vi "ResonanceAnalyzer_for_week7.vi"() -> ()   [LabVIEW 2014]
uses:
  <vilib>/imath/engines/lvmath/Plug In/_Char/NIMS_CH_character datatype.ctl
  <vilib>/imath/engines/lvmath2/RunTimeEngine/Managers/WorkSpace/UID Generator.vi
  <vilib>/imath/engines/lvmath2/RunTimeEngine/RunTimeType/NIMS_RunTimeType_From StrictType (excl LVString).vi
  <instcachedir>/0/NIMS_RunTimeType_From StrictType (excl LVString)_15A5391EEA9C4AACB9955AC755B83D29.lvgen/NIMS_RunTimeType_From StrictType (excl LVString)_15A5391EEA9C4AACB9955AC755B83D29_000.vi
  <vilib>/imath/engines/lvmath2/RunTimeEngine/LocalVariableDefStatement/MC_LocalVariableDefStatement_Display.vi
  <vilib>/imath/engines/lvmath2/RunTimeEngine/BuiltInFunctions/int32/NIMS_int32(real).vi
  <instcachedir>/0/NIMS_int32(real)_9F6AE75EF4BE45429513317A1C5A7040.lvgen/NIMS_int32(real)_9F6AE75EF4BE45429513317A1C5A7040_000.vi
  <vilib>/imath/engines/lvmath2/RunTimeEngine/BuiltInFunctions/linramp/NIMS_linramp.vi
  <vilib>/imath/engines/lvmath2/RunTimeEngine/RangeToken/NIMS_Range_R2 - Integer.vi
  <instcachedir>/0/NIMS_Range_R2 - Integer_2D1304BAF97744E0A293025746CBADFC.lvgen/NIMS_Range_R2 - Integer_2D1304BAF97744E0A293025746CBADFC_000.vi
  <vilib>/imath/engines/lvmath2/RunTimeEngine/CommandStatement/MC_CommandStatement_break.vi
  <vilib>/imath/engines/lvmath2/RunTimeEngine/IndexRead/NIMS V(S).vi
  <instcachedir>/0/NIMS V(S)_0488751826AF41519A22953C041130DC.lvgen/NIMS V(S)_0488751826AF41519A22953C041130DC_000.vi
  <vilib>/imath/engines/lvmath2/RunTimeEngine/IndexReplace/NIMS V(S)=S.vi
  <instcachedir>/0/NIMS V(S)=S_2D52C4EC15D8415E870AEE69FB516CCA.lvgen/NIMS V(S)=S_2D52C4EC15D8415E870AEE69FB516CCA_001.vi
  <vilib>/imath/engines/lvmath2/RunTimeEngine/ErrorHandling/NIMS_Create Error From Enums.vi
  <vilib>/imath/engines/lvmath/Plug In/_Char/NIMS_CH_Character RV to String.vi
  <instcachedir>/0/NIMS V(S)_0488751826AF41519A22953C041130DC.lvgen/NIMS V(S)_0488751826AF41519A22953C041130DC_003.vi
  <vilib>/imath/engines/lvmath2/RunTimeEngine/BuiltInFunctions/random/NIMS_random.vi
  <vilib>/imath/engines/lvmath2/RunTimeEngine/IndexReplace/NIMS V(S)=M.vi
  <instcachedir>/0/NIMS V(S)=M_608EF2A6197B4B6A9CB600D58D177061.lvgen/NIMS V(S)=M_608EF2A6197B4B6A9CB600D58D177061_001.vi
  <vilib>/imathl/engines/lvmath/Functions/Error Handling/Create Error.vi
  <vilib>/imath/engines/lvmath2/RunTimeEngine/BuiltInFunctions/and/NIMS_and.vi
  <instcachedir>/0/NIMS_and_04EBB299D59649339AD86944E4B9B28A.lvgen/NIMS_and_04EBB299D59649339AD86944E4B9B28A_000.vi
  <vilib>/imath/engines/lvmath/Functions/Error Handling/MergeErrorsWrapper.vi
  <vilib>/imath/engines/lvmath2/RunTimeEngine/Managers/SymbolTable/Clear UID.vi
  <vilib>/imath/engines/lvmath2/RunTimeEngine/NodeEndStatement/NIMS_NodeEndStatement_Output.vi
  <instcachedir>/0/NIMS_NodeEndStatement_Output_53EC0D466D134D7ABD903AC30B43404B.lvgen/NIMS_NodeEndStatement_Output_53EC0D466D134D7ABD903AC30B43404B_001.vi
  <instcachedir>/0/NIMS_NodeEndStatement_Output_53EC0D466D134D7ABD903AC30B43404B.lvgen/NIMS_NodeEndStatement_Output_53EC0D466D134D7ABD903AC30B43404B_010.vi
  <instcachedir>/0/NIMS_NodeEndStatement_Output_53EC0D466D134D7ABD903AC30B43404B.lvgen/NIMS_NodeEndStatement_Output_53EC0D466D134D7ABD903AC30B43404B_000.vi
  <instcachedir>/0/NIMS_NodeEndStatement_Output_53EC0D466D134D7ABD903AC30B43404B.lvgen/NIMS_NodeEndStatement_Output_53EC0D466D134D7ABD903AC30B43404B_005.vi
  <vilib>/imath/engines/lvmath2/RunTimeEngine/ErrorHandling/NIMS_Finalize Error.vi
  <vilib>/Utility/file.llb/Read From Spreadsheet File (DBL).vi
  <vilib>/imath/engines/lvmath2/RunTimeEngine/BuiltInFunctions/length/NIMS_length(GV).vi
  <instcachedir>/0/NIMS_length(GV)_08A3D13377FD4E4B96F5795FBF3698FA.lvgen/NIMS_length(GV)_08A3D13377FD4E4B96F5795FBF3698FA_000.vi
  <vilib>/imath/engines/lvmath2/RunTimeEngine/CommandStatement/NIMS_CommandStatement_MaskErr.vi
  <vilib>/imath/engines/lvmath2/RunTimeEngine/IndexRead/NIMS V(R2).vi
  <instcachedir>/0/NIMS V(R2)_C76619605A0E4E9F8B2FA9389712AC47.lvgen/NIMS V(R2)_C76619605A0E4E9F8B2FA9389712AC47_000.vi
  <vilib>/imath/engines/lvmath2/RunTimeEngine/Managers/SymbolTable/NIMS_WorkSpace.lvlib
panel:
  out "Non Lin Coefficients \n(Amp, Q fac, Center Freq)":dbl[](array[numeric])=[2.8103706495498373, 25.122070589973074, 18.455137765578083]
  out "residual":dynamicdata(graph)=[{"t0"=timestamp(0 s since 1904-01-01), "dt"=1.0, "Y"=[-0.010626904483554396, 0.006405074216437016, 0.014962795381668715, -0.0007789639875173861, -0.010040446965700117], "attributes"=variant("NI_ChannelName"=variant(string "Residual"))}]
  out "Fit graph using coefficients":dynamicdata(graph)=[{"t0"=timestamp(0 s since 1904-01-01), "dt"=1.0, "Y"=[0.013975044483554395, 0.013511065783562983, 0.013077284618331284, 0.012670813987517387, 0.012289126965700116], "attributes"=variant("NI_ChannelName"=variant(string "Best fit"))}]
  out "Results":T1={"Q 2"=16.0, "Amp"=0.02804008, "Max Frequency"=160.0}
  out "newFreq vs newAmp":cluster{"Freq":dbl[], "Amp":dbl[]}(graph)={"Freq"=[150.0, 155.0, 160.0, 165.0, 170.0], "Amp"=[0.00334814, 0.01991614, 0.02804008, 0.01189185, 0.00224868]}
  in  "Tab Control":enum32{"Simulation", "Experiment"}(tab)=enum."Experiment"
  in  "Center Frequency":dbl=600.0
  in  "Q":dbl=10.0
  in  "Start Frequency":dbl=400.0
  in  "End Frequency":dbl=800.0
  in  "df":dbl=5.0
  in  "Noise Level":dbl=0.003
  in  "Path":path=path "C:/Users/josephds/Desktop/my_week7/week7/data.txt"
  out "Freq and Gain Array":dbl[][](array[numeric])=[[0.0, 5.0, 10.0, 15.0, 20.0, 25.0, 30.0, 35.0, 40.0, 45.0, 50.0, 55.0, 60.0, 65.0, 70.0, 75.0, 80.0, 85.0, 90.0, 95.0, 100.0, 105.0, 110.0, 115.0, 120.0, 125.0, 130.0, 135.0, 140.0, 145.0, 150.0, 155.0, 160.0, 165.0, 170.0, 175.0, 180.0, 185.0, 190.0, 195.0, 200.0, 205.0, 210.0, 215.0, 220.0, 225.0, 230.0, 235.0, 240.0, 245.0, 250.0, 255.0, 260.0, 265.0, 270.0, 275.0, 280.0, 285.0, 290.0, 295.0, 300.0, 305.0, 310.0, 315.0, 320.0, 325.0, 330.0, 335.0, 340.0, 345.0, 350.0, 355.0, 360.0, 365.0, 370.0, 375.0, 380.0, 385.0, 390.0, 395.0, 400.0, 405.0, 410.0, 415.0, 420.0, 425.0, 430.0, 435.0, 440.0, 445.0, 450.0, 455.0, 460.0, 465.0, 470.0, 475.0, 480.0, 485.0, 490.0, 495.0], [0.00012746, 0.00019638, 0.0006129, 0.0018897, 0.00197803, 0.00073736, 0.000241, 0.00029292, 0.00016885, 5.355e-05, 9.619e-05, 6.145e-05, 0.00015307, 9.994e-05, 6.054e-05, 1.069e-05, 4.57e-05, 1.057e-05, 3.062e-05, 5.58e-05, 0.00012394, 0.00014636, 5.86e-05, 0.00044327, 0.0007657, 0.00048589, 0.0001038, 0.00029858, 0.00114892, 0.00365701, 0.00334814, 0.01991614, 0.02804008, 0.01189185, 0.00224868, 0.00039642, 0.00255818, 0.00233139, 0.00068615, 7.402e-05, 2.625e-05, 8.296e-05, 2.457e-05, 3.326e-05, 4.624e-05, 7.794e-05, 4.182e-05, 4.962e-05, 9.364e-05, 8.061e-05, 5.068e-05, 3.313e-05, 2.052e-05, 8.053e-05, 0.00010256, 9.34e-06, 5.71e-05, 0.00010789, 8.744e-05, 6.621e-05, 9.243e-05, 0.0002253, 0.00131791, 0.00295714, 0.00403, 0.00331379, 0.00129275, 0.00035791, 0.00218109, 0.0036526, 0.00305069, 0.00198481, 0.0007002, 0.00042371, 0.00013887, 3.3e-05, 5.2e-05, 0.00011501, 1.843e-05, 1.444e-05, 2.425e-05, 2.039e-05, 4.973e-05, 2.103e-05, 2.497e-05, 2.991e-05, 7.599e-05, 8.205e-05, 5.579e-05, 0.00013745, 0.0001572, 7.003e-05, 9.92e-05, 0.00010997, 0.00028432, 0.00068847, 0.00122175, 0.00130637, 0.00136855, 0.00095653]] format="%0.3f"
  out "max":dbl=0.02804008
  out "min":dbl=9.34e-06
  # "NOTE: x scale is in Time instead of Frequency"
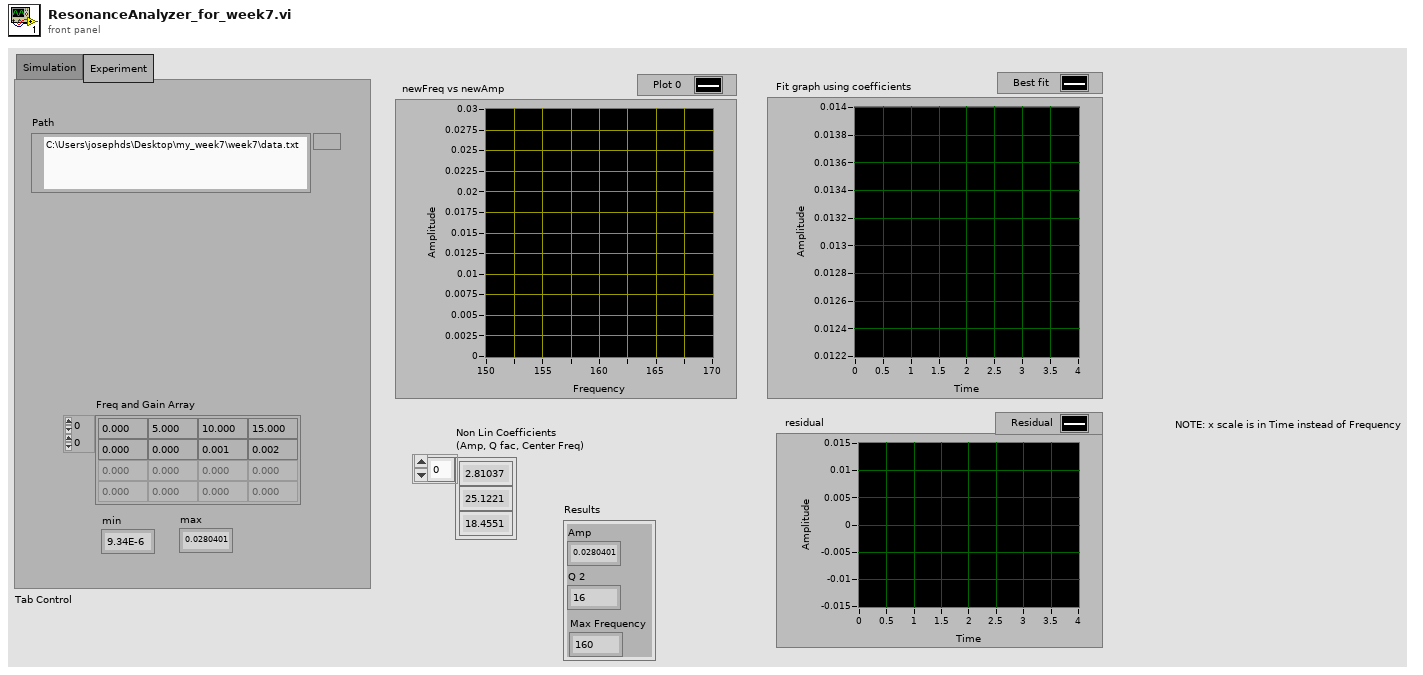
[diagram p1: front panel]
types:
  T1 = cluster{"Q 2":dbl, "Amp":dbl, "Max Frequency":dbl}
  T2 = typedef "NIMS_CH_character datatype.ctl" = cluster{"Numeric":u8}
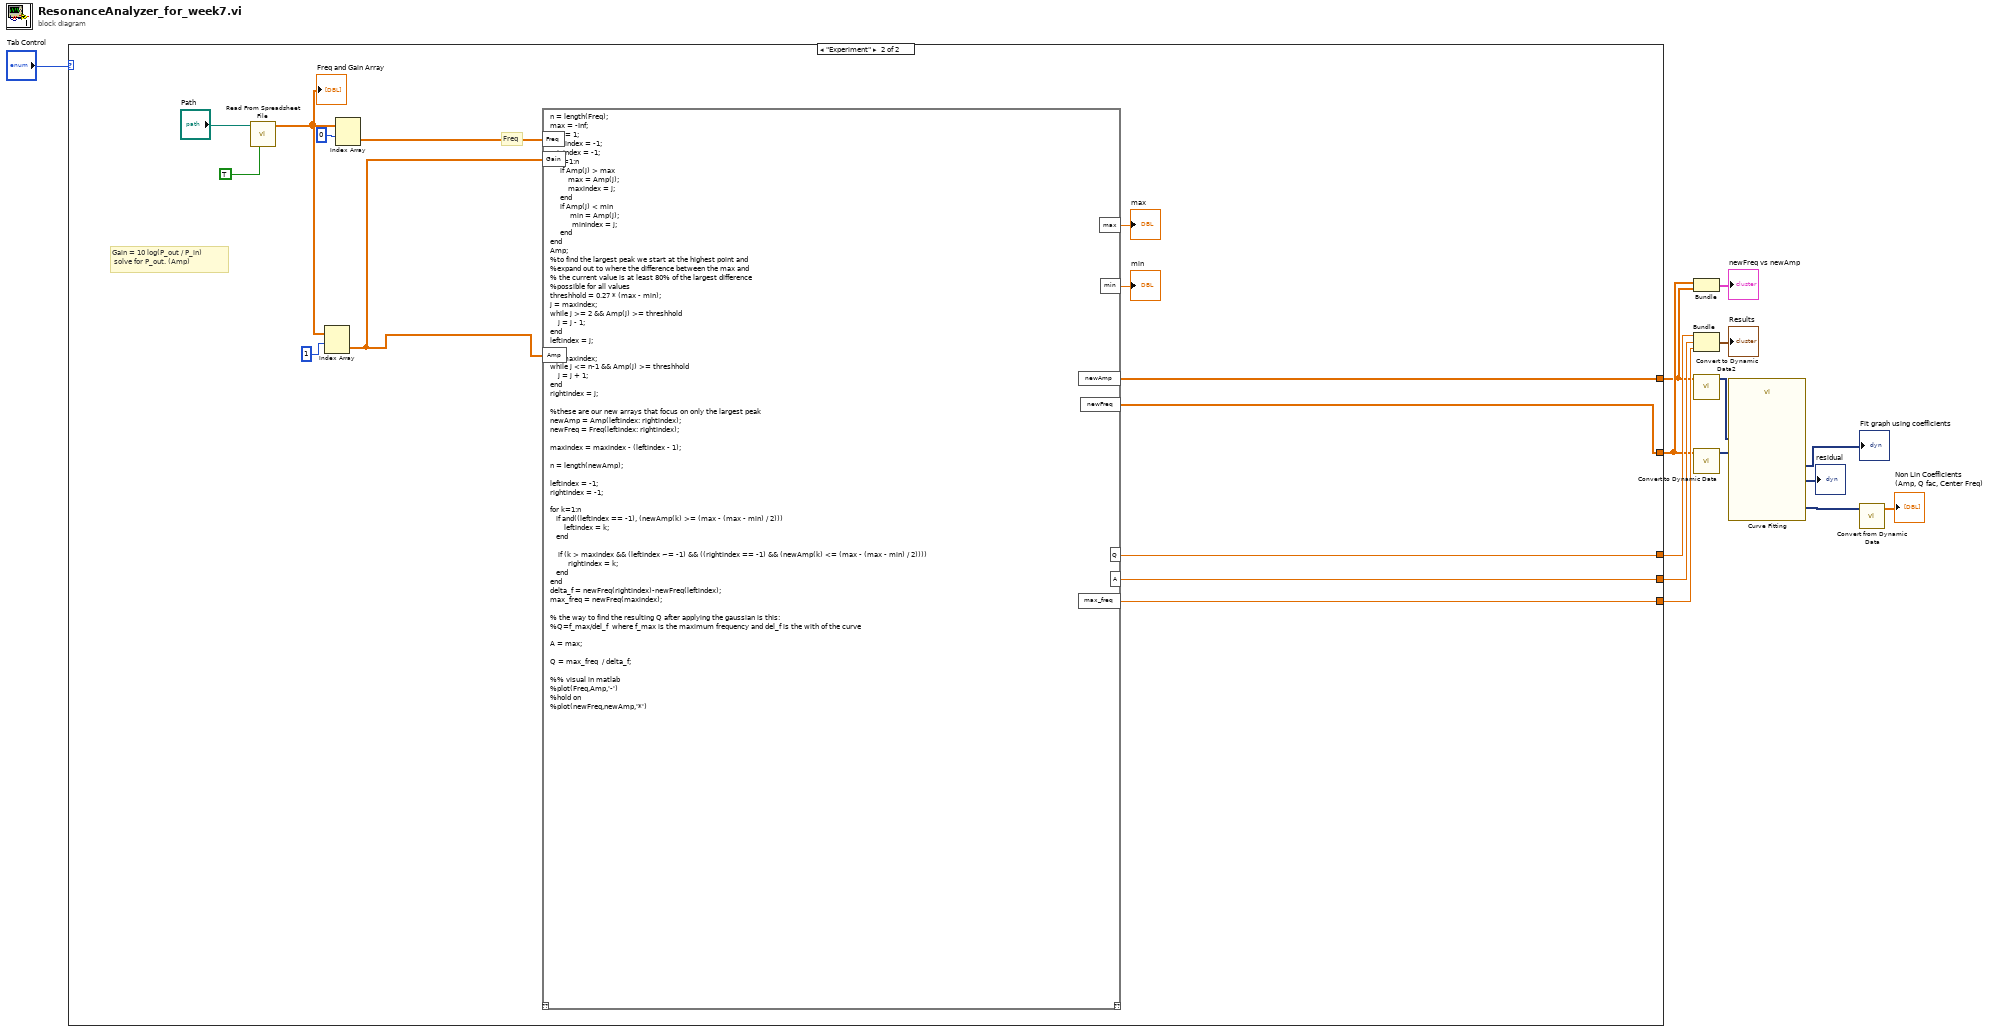
[diagram p0: block diagram]
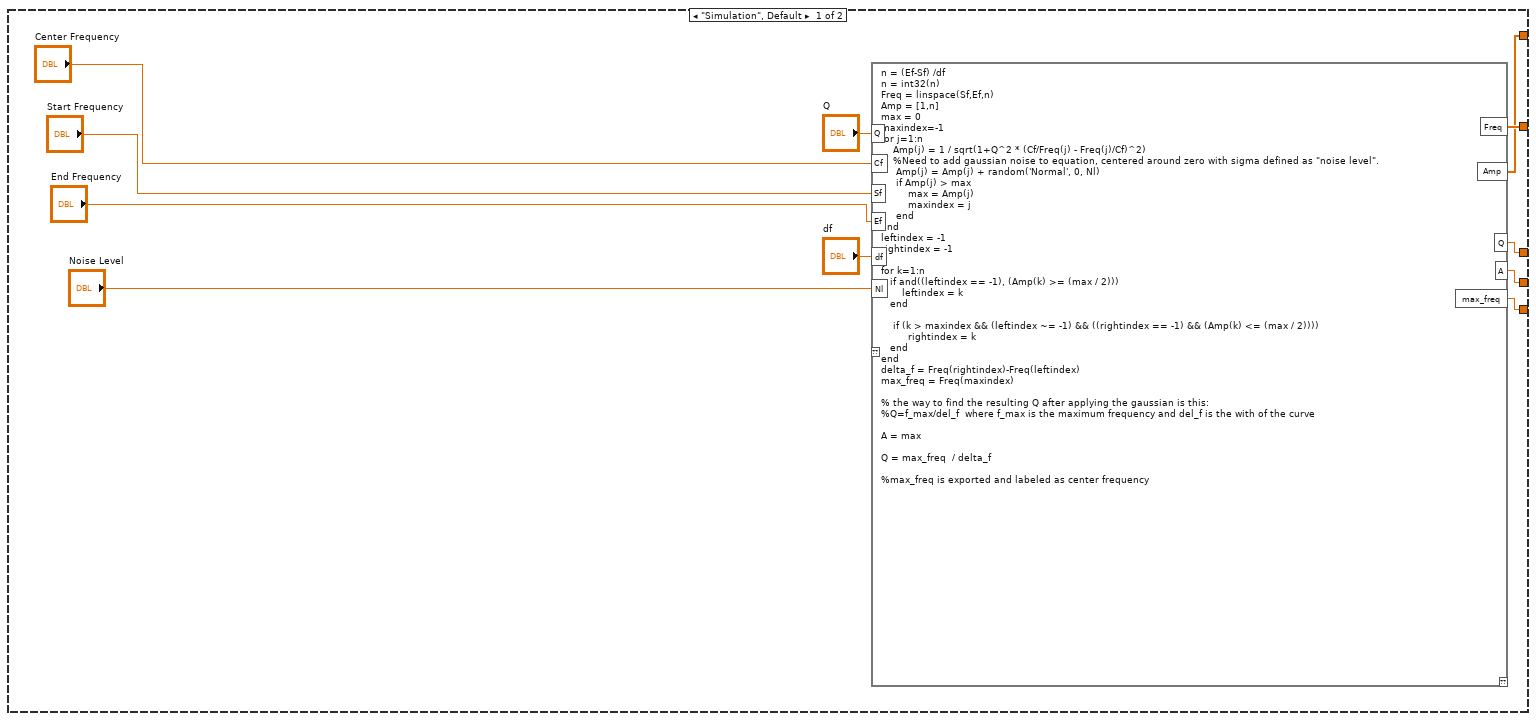
[diagram p2: hidden frame]
diagram:
  n1 = case shown="\"Experiment\"" "Tab Control" {
    tunnel: [w19 w675] -> w8
    tunnel: [w18 w676] -> w5
    tunnel: [w17 w674] -> w12
    tunnel: [w16 w673] -> w11
    tunnel: [w15 w672] -> w10
    frame "Simulation", Default {
      n2 = mathscript code="n = (Ef-Sf) /df\nn = int32(n)\nFreq = linspace(Sf,Ef,n)\nAmp = [1,n]\nmax = 0\nmaxindex=-1\nfor j=1:n\n    Amp(j) = 1 / sqrt(1+Q^2 * (Cf/Freq(j) - Freq(j)/Cf)^2)\n    %Need to add gaussian noise to equation, centered around zero with sigma defined as \"noise level\".\n     Amp(j) = Amp(j) + random('Normal', 0, Nl)\n     if Amp(j) > max\n         max = Amp(j)\n         maxindex = j\n     end\nend\nleftindex = -1\nrightindex = -1\n\nfor k=1:n\n   if and((leftindex == -1), (Amp(k) >= (max / 2)))\n       leftindex = k\n   end\n\n    if (k > maxindex && (leftindex ~= -1) && ((rightindex == -1) && (Amp(k) <= (max / 2))))\n         rightindex = k\n   end\nend\ndelta_f = Freq(rightindex)-Freq(leftindex)\nmax_freq = Freq(maxindex)\n\n% the way to find the resulting Q after applying the gaussian is this:\n%Q=f_max/del_f  where f_max is the maximum frequency and del_f is the with of the curve \n\nA = max\n\nQ = max_freq  / delta_f\n\n%max_freq is exported and labeled as center frequency"("Q"="Q", "Cf"="Center Frequency", "Sf"="Start Frequency", "Ef"="End Frequency", "df"="df", "Nl"="Noise Level") -> ("Freq"=w19:dbl[], "Amp"=w18:cdb[], "Q"=w17:dbl, "A"=w16:cdb, "max_freq"=w15:dbl)  [unwired: 1 in, 1 out]
    }
    frame "Experiment" {
      # "Gain = 10 log(P_out / P_in)\n solve for P_out. (Amp)"
      # "Freq"
      n3 = call-poly <vilib>:"Read From Spreadsheet File.vi"("transpose (no:F)"=TRUE, "file path (dialog if empty)"="Path") -> ("all rows"=w681:dbl[][])  [unwired: 5 in, 4 out]
      "Freq and Gain Array" <- w681
      n4 = Index Array(array=w681, index (row)=1) -> (element=w671:dbl[])  [unwired: 1 in]
      n5 = Index Array(array=w681, index (row)=0) -> (element=w679:dbl[])  [unwired: 1 in]
      n6 = mathscript code="n = length(Freq);\nmax = -Inf;\nmin = 1;\nmaxindex = -1;\nminindex = -1;\nfor j=1:n\n     if Amp(j) > max\n         max = Amp(j);\n         maxindex = j;\n     end\n     if Amp(j) < min\n          min = Amp(j);\n           minindex = j;\n     end\nend\nAmp;\n%to find the largest peak we start at the highest point and\n%expand out to where the difference between the max and \n% the current value is at least 80% of the largest difference \n%possible for all values \nthreshhold = 0.27 * (max - min);\nj = maxindex;\nwhile j >= 2 && Amp(j) >= threshhold\n    j = j - 1;\nend\nleftindex = j;\n\nj = maxindex;\nwhile j <= n-1 && Amp(j) >= threshhold\n    j = j + 1;\nend\nrightindex = j;\n\n%these are our new arrays that focus on only the largest peak\nnewAmp = Amp(leftindex: rightindex);\nnewFreq = Freq(leftindex: rightindex);\n\nmaxindex = maxindex - (leftindex - 1);\n\nn = length(newAmp);\n\nleftindex = -1;\nrightindex = -1;\n\nfor k=1:n\n   if and((leftindex == -1), (newAmp(k) >= (max - (max - min) / 2)))\n       leftindex = k;\n   end\n\n    if (k > maxindex && (leftindex ~= -1) && ((rightindex == -1) && (newAmp(k) <= (max - (max - min) / 2))))\n         rightindex = k;\n   end\nend\ndelta_f = newFreq(rightindex)-newFreq(leftindex);\nmax_freq = newFreq(maxindex);\n\n% the way to find the resulting Q after applying the gaussian is this:\n%Q=f_max/del_f  where f_max is the maximum frequency and del_f is the with of the curve \n\nA = max;\n\nQ = max_freq  / delta_f;\n\n%% visual in matlab\n%plot(Freq,Amp,'-')\n%hold on\n%plot(newFreq,newAmp,'*')"("Freq"=w679, "Gain"=w671, "Amp"=w671) -> ("max"=→"max":dbl, "min"=→"min":dbl, "newAmp"=w676:dbl[], "newFreq"=w675:dbl[], "Q"=w674:dbl, "A"=w673:dbl, "max_freq"=w672:dbl)  [unwired: 1 in, 1 out]
    }
  }
  n7 = Bundle("newFreq"=w8, "Amp"=w5) -> (→"newFreq vs newAmp":cluster{"newFreq":dbl[], "Amp":cdb[]})  [unwired: 1 in]
  n8 = Bundle("Q"=w12, "A"=w11, "max_freq"=w10) -> (→"Results":cluster{"Q":dbl, "A":cdb, "max_freq":dbl})  [unwired: 1 in]
  n9 = call "Convert to Dynamic Data2"("Array"=w5) -> ("Dynamic Data Type"=w6:dynamicdata)  [unwired: 3 in]
  n10 = call "Convert to Dynamic Data"("Array"=w8) -> ("Dynamic Data Type"=w7:dynamicdata)  [unwired: 3 in]
  n11 = call "Curve Fitting"("Locations"=w7, "Signals"=w6) -> ("residual"=→"residual":dynamicdata, "best fit"=→"Fit graph using coefficients":dynamicdata, "non-linear coefficients"=w4:dynamicdata)  [unwired: 5 in, 2 out]
  n12 = call "Convert from Dynamic Data"("Dynamic Data Type"=w4) -> ("Array"=→"Non Lin Coefficients \n(Amp, Q fac, Center Freq)":dbl[])  [unwired: 3 in]
